vi "Parse Cluster Ref.vi"(11 "Cluster Ref":refnum<vi>) -> (3 "Controls Refs and Types":T1)   [LabVIEW 2020, in "DQMH_API.lvlib"]
uses:
  DQMH_API.lvlib
  Controls Refs and Type--cluster.ctl
  <vilib>/Utility/Data Type/Type Definitions/Data Type.ctl
  <vilib>/Utility/Data Type/NI_Data Type.lvlib
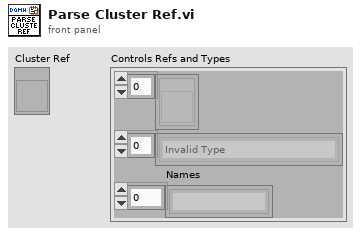
[diagram p1: front panel]
types:
  T1 = typedef "DQMH_API.lvlib/Controls Refs and Type--cluster.ctl" = cluster{"Ctrls Refs ":refnum<vi>[], "Ctrls Types":T2[], "Names":string[]}
  T2 = typedef "NI_Data Type.lvlib/Data Type.ctl" = enum8{"Invalid Type", "Void", "I8", "I16", "I32", "I64", "U8", "U16", "U32", "U64", "Single Float", "Double Float", "Extended Float", "Single Complex", "Double Complex", "Extended Complex", "Enum U8", "Enum U16", "Enum U32", "Enum U64", "Single Float With Unit", "Double Float With Unit", "Extended Float With Unit", "Single Complex with Unit", "Double Complex with Unit", "Extended Complex with Unit", "Boolean", "String", "Path", "Picture", "Tag", "Array", "Cluster", "Variant", "LV Variant", "Waveform", "Timestamp", "Digital Waveform", "Digital Data", "ExpressData", "Refnum", "External Data", "VI", "Poly VI", "LabVIEW Class Instance", "Fixed Point", "Set Collection", "Map Collection"}
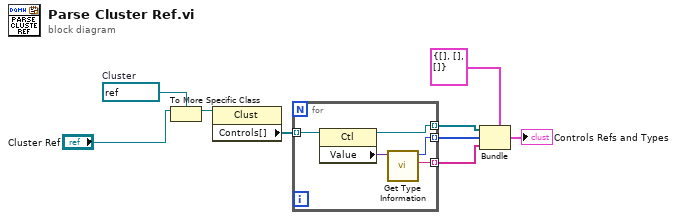
[diagram p0: block diagram]
diagram:
  w7 = refnum<vi> refnum  # Cluster
  n1 = To More Specific Class(target class=w7, reference="Cluster Ref") -> (specific class reference=w8:refnum<vi>)  [unwired: 1 in, 1 out]
  n2 = property class="Clust"(reference=w8) -> ("Controls[]"=w6:refnum<vi>[])  [unwired: 1 in, 2 out]
  n3 = for {
    tunnel: w6 -> [w14] mode=indexing
    tunnel: [w12] -> w5 mode=indexing
    tunnel: [w11] -> w2 mode=indexing
    tunnel: [w10] -> w1 mode=indexing
    n4 = property class="Ctl"(reference=w14) -> (reference out=w12:refnum<vi>, "Value"=w13:variant)  [unwired: 1 in, 1 out]
    n5 = call <vilib>:"Get Type Information.vi"("variant"=w13) -> ("name"=w10:string, "type"=w11:T2)  [unwired: 6 in, 3 out]
  }
  n6 = Bundle(cluster=T1 {"Ctrls Refs "=[], "Ctrls Types"=[], "Names"=[]} ("Indicators"), "Ctrls Refs"=w5, "Ctrls Types"=w2, "Names"=w1) -> (→"Controls Refs and Types":T1)
